vi "Write Output.vi"(8 "error in (no error)":errorcluster, 10 "Output":refnum<k21>, 11 "TestMPU in":refnum<class "TestMPU.lvclass">) -> (0 "error out":errorcluster, 3 "TestMPU out":refnum<class "TestMPU.lvclass">)   [LabVIEW 2018]
uses:
  TestMPU.lvclass
  C:/Users/pkubanek/ts_m1m3thermalFPGA/src/Modbus_Processing_Unit/src/MPU.lvclass
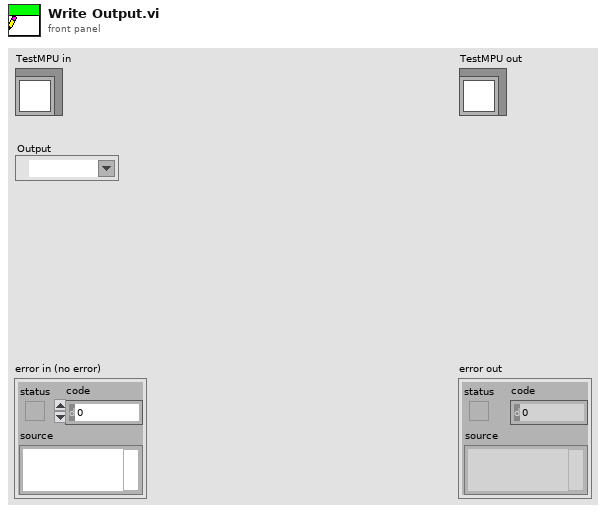
[diagram p1: front panel]
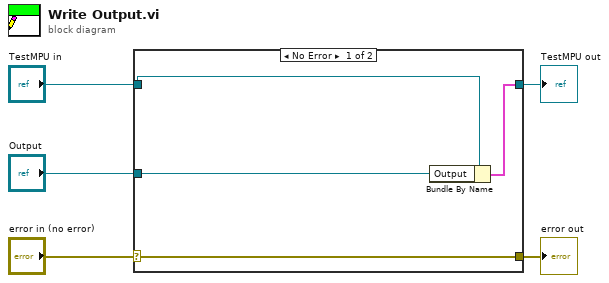
[diagram p0: block diagram]
diagram:
  n1 = case shown="No Error" "error in (no error)" {
    selector: "error in (no error)" -> [w9 w10]
    tunnel: [w9 w10] -> w4
    tunnel: [w7 w11] -> w2
    tunnel: "TestMPU in" -> [w8 w11]
    tunnel: "Output" -> [w6 _]
    frame No Error {
      n2 = Bundle By Name(cluster=w8, "Output"=w6) -> (w7:cluster{})
    }
    frame Error {
    }
  }
  "error out" <- w4
  "TestMPU out" <- w2
